vi "eWriteNames and eReadNames with Open.vi"(5 "aWriteValues":dbl[](array[numeric]) format="%.2f", 6 "aReadNames":string[](array[string]), 7 "aWriteNames":string[](array[string]), 8 "error in":errorcluster, 9 "Identifier":string="LJM_idANY", 10 "ConnectionType":string="LJM_ctANY", 11 "DeviceType":string="LJM_dtANY") -> (0 "error out":errorcluster, 3 "Handle Out":i32, 4 "aReadValues":dbl[](array[numeric]) format="%.2f")   [LabVIEW 2024]
panel:
  out "Error String":string
  # "Usually we like to call open in the main VI and then pass the handle around to sub-vis,\nbut this VI includes an Open call so it can be called without any prior calls.  When you\ndo a repeat Open call that would result in a handle to an already open device that Open\ncall just returns that already active handle again, so repeat Open calls are no problem and\nreally take no time.  Also, this VI does not call Close so can be used in parallel code.\n\nThis utility VI does 2 LJM calls ... a call to eReadNames followed by a call to\neWriteNames ... which will result in at least 2 low-level modbus transactions.  This can\nbe done more efficiently with eNames which will use 1 modbus transaction if\npossible, but this utility VI might be a simpler option when max speed is not important."
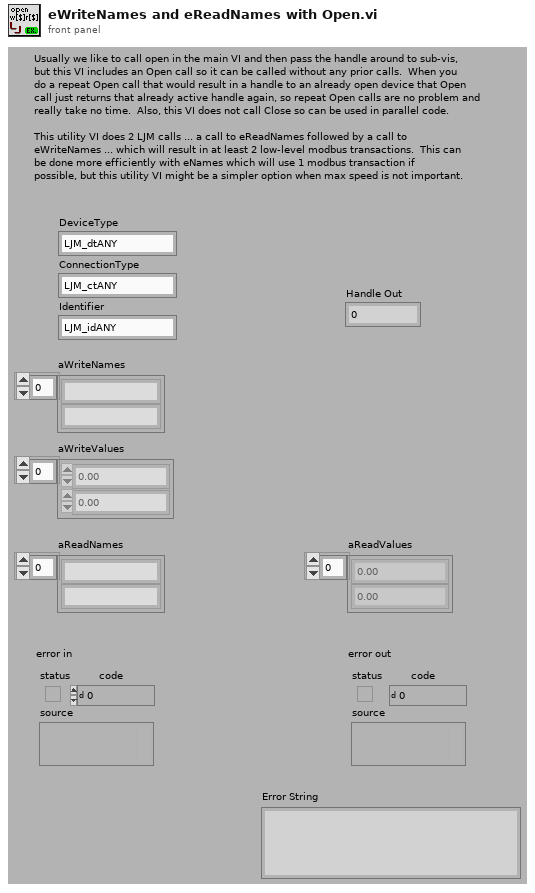
[diagram p1: front panel]
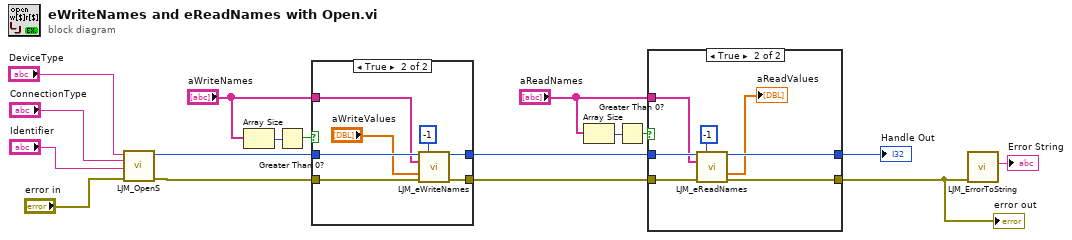
[diagram p0: block diagram]
diagram:
  n1 = call "LJM_OpenS.vi"("error in"="error in", "Identifier"="Identifier", "ConnectionType"="ConnectionType", "DeviceType"="DeviceType") -> ("error out"=w5:errorcluster, "Handle"=w1:i32)  [unwired: 6 in]
  n2 = Array Size(array="aWriteNames") -> (size(s)=w11:i32)
  n3 = Greater Than 0?(x=w11) -> (x > 0?=w12:bool)
  n4 = case shown="True" w12 {
    tunnel: w1 -> [w19 w26]
    tunnel: w5 -> [w18 w25]
    tunnel: [w18 w24] -> w16
    tunnel: [w19 w23] -> w15
    tunnel: "aWriteNames" -> [_ w22]
    frame False {
    }
    frame True {
      n5 = call "LJM_eWriteNames.vi"("Handle In"=w26, "NumFrames (Auto-Detect)"=-1, "aNames"=w22, "aValuesIn"="aWriteValues", "error in"=w25) -> ("Handle Out"=w23:i32, "error out"=w24:errorcluster)  [unwired: 8 in, 1 out]
    }
  }
  n6 = Array Size(array="aReadNames") -> (size(s)=w9:i32)
  n7 = Greater Than 0?(x=w9) -> (x > 0?=w7:bool)
  n8 = case shown="True" w7 {
    tunnel: w16 -> [w27 w35]
    tunnel: w15 -> [w28 w34]
    tunnel: [w28 w33] -> w14
    tunnel: [w27 w32] -> w13
    tunnel: "aReadNames" -> [_ w31]
    frame False {
    }
    frame True {
      n9 = call "LJM_eReadNames.vi"("Handle In"=w34, "NumFrames (Auto-Detect)"=-1, "aNames"=w31, "error in"=w35) -> ("Handle Out"=w33:i32, "aValuesOut"=→"aReadValues":dbl[], "error out"=w32:errorcluster)  [unwired: 8 in, 1 out]
    }
  }
  "error out" <- w13
  "Handle Out" <- w14
  n10 = call "LJM_ErrorToString.vi"("error in"=w13) -> ("String"=→"Error String":string)  [unwired: 10 in]
